vi "robot_main.vi"(11 "input string":string) -> (2 "count?":bool, 3 "output string":string)   [LabVIEW 2020]
uses:
  status/filter_vial_No.vi
  Robot-HL/small_scara_interface/small_scara_interface.lvlib
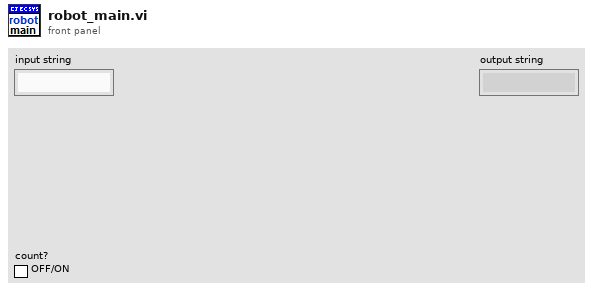
[diagram p1: front panel]
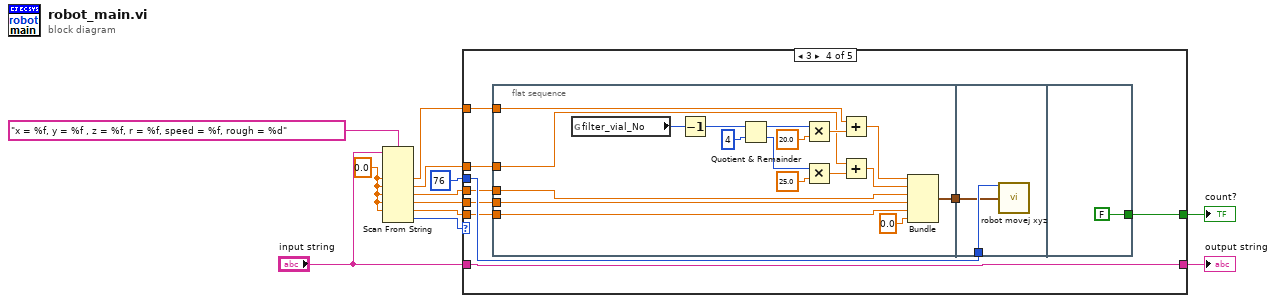
[diagram p0: block diagram]
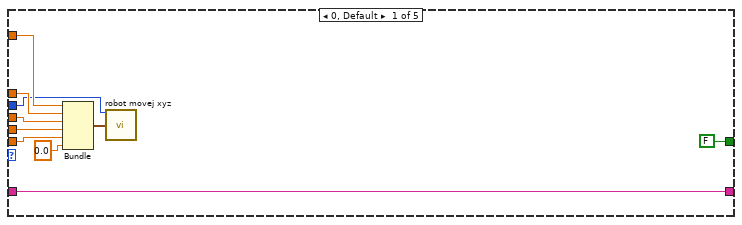
[diagram p2: hidden frame]
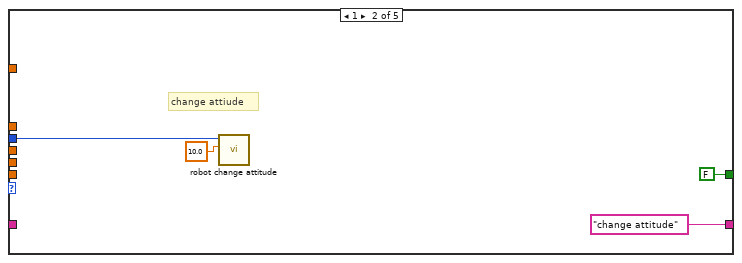
[diagram p3: hidden frame]
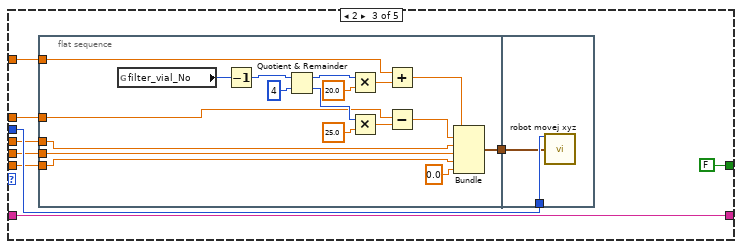
[diagram p4: hidden frame]
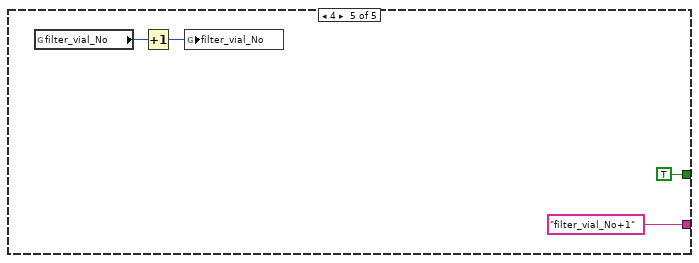
[diagram p5: hidden frame]
diagram:
  w6 = sgl 0.0
  n1 = Scan From String(format string="x = %f, y = %f , z = %f, r = %f, speed = %f, rough = %d", input string="input string", default 1=w6, default 2=w6, default 3=w6, default 4=w6, default 5=w6) -> (output 1=w11:sgl, output 2=w10:sgl, output 3=w9:sgl, output 4=w8:sgl, output 5=w7:sgl, output 6=w5:i32)  [unwired: 3 in, 3 out]
  n2 = case shown="3" w5 {
    tunnel: 76 ("robot_id") -> [w14 w23 w35 w63 _]
    tunnel: w11 -> [w22 _ w33 w61 _]
    tunnel: w10 -> [w21 _ w32 w60 _]
    tunnel: w9 -> [w20 _ w31 w59 _]
    tunnel: w8 -> [w19 _ w30 w58 _]
    tunnel: w7 -> [w18 _ w29 w57 _]
    tunnel: [w17 "change attitude" w28 w62 "filter_vial_No+1" ("input string")] -> w3
    tunnel: "input string" -> [w17 _ w28 w62 _]
    tunnel: [FALSE ("count?") FALSE ("count?") FALSE ("count?") w56 TRUE ("count?")] -> w1
    frame 0, Default {
      n3 = Bundle(w22, w21, w20, w19, w18, sgl 0.0) -> (w13:cluster{sgl, sgl, sgl, sgl, sgl, sgl})  [unwired: 1 in]
      n4 = call "robot movej xyz.vi"("robot_id"=w14, "参数"=w13) -> ()  [unwired: 12 in, 2 out]
    }
    frame 1 {
      # "change attiude"
      n5 = call "robot change attitude.vi"("float speed"=sgl 10.0, "robot_id"=w23) -> ()  [unwired: 9 in, 1 out]
    }
    frame 2 {
      n6 = flat-sequence {
        tunnel: [w41] -> w34
        tunnel: w33 -> [w40]
        tunnel: w32 -> [w39]
        tunnel: w31 -> [w38]
        tunnel: w30 -> [w37]
        tunnel: w29 -> [w36]
        tunnel: w35 -> [w55]
        tunnel: w34 -> [w54]
        frame #0 {
          n7 = global read "filter_vial_No.vi" "filter_vial_No"() -> (w49:i32)
          n8 = Decrement(x=w49) -> (x-1=w48:i32)
          n9 = Quotient & Remainder(x=w48, y=4) -> (x-y*floor(x/y)=w51:i32, floor(x/y)=w50:i32)
          n10 = Multiply(x=w51, y=sgl 20.0) -> (x*y=w52:sgl)
          n11 = Multiply(x=w50, y=sgl 25.0) -> (x*y=w43:sgl)
          n12 = Add(x=w40, y=w52) -> (x+y=w53:sgl)
          n13 = Subtract(x=w39, y=w43) -> (x-y=w42:sgl)
          n14 = Bundle(w53, w42, w38, w37, w36, "rough"=sgl 0.0) -> (w41:cluster{sgl, sgl, sgl, sgl, sgl, "rough":sgl})  [unwired: 1 in]
        }
        frame #1 {
          n15 = call "robot movej xyz.vi"("robot_id"=w55, "参数"=w54) -> ()  [unwired: 12 in, 2 out]
        }
      }
    }
    frame 3 {
      n16 = flat-sequence {
        tunnel: [w72] -> w64
        tunnel: w61 -> [w71]
        tunnel: w60 -> [w65]
        tunnel: w59 -> [w70]
        tunnel: w58 -> [w69]
        tunnel: w57 -> [w68]
        tunnel: w64 -> [w83]
        tunnel: w63 -> [w84]
        tunnel: [FALSE ("count?")] -> w56
        frame #0 {
          n17 = global read "filter_vial_No.vi" "filter_vial_No"() -> (w78:i32)
          n18 = Decrement(x=w78) -> (x-1=w77:i32)
          n19 = Quotient & Remainder(x=w77, y=4) -> (x-y*floor(x/y)=w80:i32, floor(x/y)=w79:i32)
          n20 = Multiply(x=w80, y=sgl 20.0) -> (x*y=w81:sgl)
          n21 = Multiply(x=w79, y=sgl 25.0) -> (x*y=w66:sgl)
          n22 = Add(x=w71, y=w81) -> (x+y=w82:sgl)
          n23 = Add(x=w65, y=w66) -> (x+y=w67:sgl)
          n24 = Bundle(w82, w67, w70, w69, w68, "rough"=sgl 0.0) -> (w72:cluster{sgl, sgl, sgl, sgl, sgl, "rough":sgl})  [unwired: 1 in]
        }
        frame #1 {
          n25 = call "robot movej xyz.vi"("robot_id"=w84, "参数"=w83) -> ()  [unwired: 12 in, 2 out]
        }
        frame #2 {
        }
      }
    }
    frame 4 {
      n26 = global read "filter_vial_No.vi" "filter_vial_No"() -> (w89:i32)
      n27 = Increment(x=w89) -> (x+1=w88:i32)
      n28 = global write "filter_vial_No.vi" "filter_vial_No"(w88) -> ()
    }
  }
  "output string" <- w3
  "count?" <- w1
